vi "z_control_statemachine.vi"(4 "Kiz_down":sgl format="%#_13g", 6 "z_axis_params":T1={"TOL"=0.0, "ramp_rate"=-5e-06, "z_u_max"=5.0, "setpoint"=0.0, "Ki"=0.0, "Z_error_threshold"=0.0, "Z_settled_samples_threshold "=0, "z_UP"=1.5, "zup_N"=5000} {"ramp_rate" format="%#_4g"}, 7 "step_down":bool, 8 "step_down_frac":fxp<+,8,1>, 9 "init Z up":fxp<+/-,16,5>, 10 "State":i8, 11 "zerr(k)":fxp<+/-,16,5>) -> (3 "z-u(k)":fxp<+/-,16,5>)   [LabVIEW 2017]
uses:
  controls/z-axis-params_ssxy.ctl
  <vilib>/rvi/Emulation/niFpgaEmulationIsFPGAContextNoSignature.vi
  <vilib>/rvi/DataTransferAndStorage/Container/Common/niFpgaContainerGetUniqueNameForEmu.vi
  <vilib>/rvi/Memory/Memory_Emulation/niFpgaMemoryEmulationCacheClearOnFirstRun.vi
  <vilib>/rvi/Memory/Memory_Emulation/nirvimemoryEmulationManagerCache_MakeExclusive.vi
  <vilib>/rvi/Memory/Memory_Emulation/niFpgaMemoryEmulationValidateCache.vi
  <vilib>/rvi/Memory/Memory_Emulation/nirvimemoryEmulationManagerCache_InsertValue.vi
  <vilib>/Utility/error.llb/Clear Errors.vi
  <vilib>/rvi/Memory/Memory_Emulation/nirvimemoryEmulationManagerCache_ReleaseExclusive.vi
  <vilib>/rvi/Memory/Memory_Emulation/nirvimemoryEmulationManagerCache_GetValue.vi
  <vilib>/rvi/Memory/Memory_Emulation/nirvimemoryEmulationManagerCache_SetValue.vi
  <vilib>/rvi/Emulation/niFpgaProcessEmulError.vi
  <vilib>/rvi/Emulation/niFpgaSctlEmulationGetInTimedLoop.vi
  <vilib>/rvi/DataTransferAndStorage/Container/XNode/niFpgaContainer.xnode
  <vilib>/rvi/DataTransferAndStorage/Register/Emulation/niFpgaRegisterEmulation.vi
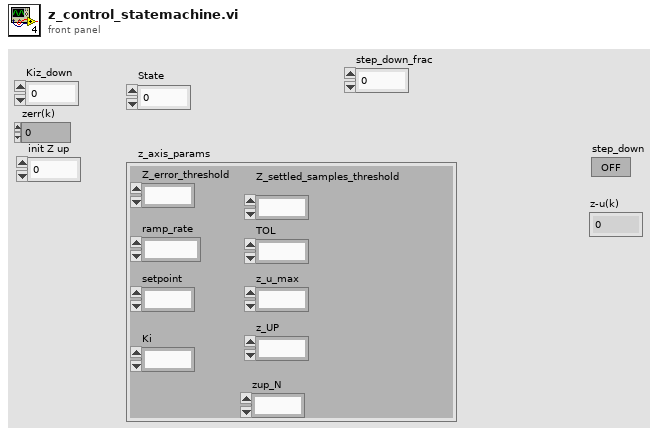
[diagram p1: front panel]
types:
  T1 = typedef "z-axis-params_ssxy.ctl" = cluster{"TOL":fxp<+/-,16,2>, "ramp_rate":sgl, "z_u_max":fxp<+/-,16,5>, "setpoint":fxp<+/-,16,5>, "Ki":fxp<+,16,1>, "Z_error_threshold":fxp<+/-,16,5>, "Z_settled_samples_threshold ":i16, "z_UP":fxp<+/-,16,5>, "zup_N":i16}
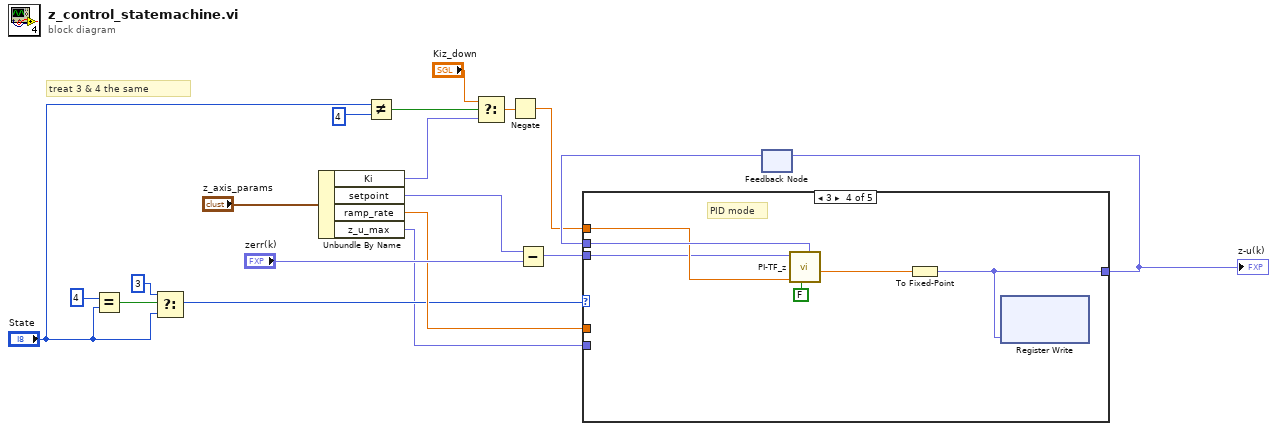
[diagram p0: block diagram]
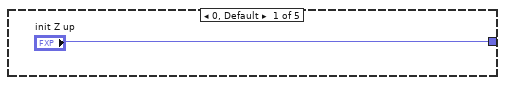
[diagram p2: hidden frame]
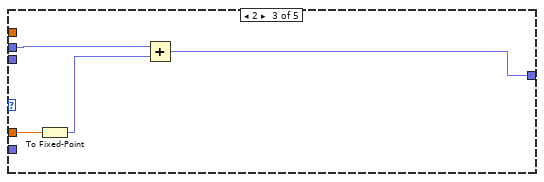
[diagram p4: hidden frame]
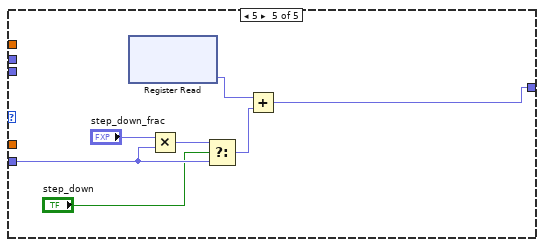
[diagram p5: hidden frame]
diagram:
  # "treat 3 & 4 the same"
  n1 = Equal?(x=i8 4 ("y"), y="State") -> (x = y?=w9:bool)
  n2 = Select(t=i8 3 ("y"), s=w9, f="State") -> (s? t:f=w7:i8)
  n3 = Unbundle By Name("z_axis_params") -> ("Ki"=w2:fxp<+,16,1>, "setpoint"=w3:fxp<+/-,16,5>, "ramp_rate"=w10:sgl, "z_u_max"=w1:fxp<+/-,16,5>)
  n4 = Not Equal?(x="State", y=i8 4) -> (x != y?=w18:bool)
  n5 = Select(t="Kiz_down", s=w18, f=w2) -> (s? t:f=w17:sgl)
  n6 = Negate(x=w17) -> (-x=w12:sgl)
  n7 = Subtract(x=w3, y="zerr(k)") -> (x-y=w11:fxp<+/-,17,6>)
  n8 = feedback #1() -> (w13:fxp<+/-,25,7>)  [unwired: 1 in]
  n9 = case shown="3" w7 {
    tunnel: ["init Z up" w21 w24 w26 w34] -> w6
    tunnel: w13 -> [_ w21 w22 w30 _]
    tunnel: w12 -> [_ _ _ w29 _]
    tunnel: w11 -> [_ _ _ w28 _]
    tunnel: w10 -> [_ _ w25 _ _]
    tunnel: w1 -> [_ _ _ _ w33]
    frame 0, Default {
    }
    frame 1 {
      # "XY-move, hold still, for now"
    }
    frame 2 {
      n10 = To Fixed-Point(number=w25) -> (fixed-point=w23:fxp<+/-,16,5>)  [unwired: 1 in]
      n11 = Add(x=w22, y=w23) -> (x+y=w24:fxp<+/-,16,5>)
    }
    frame 3 {
      # "PID mode"
      n12 = call "PI-TF_z.vi"("u(k-1)"=w30, "reset"=FALSE, "Ki"=w29, "e(k)"=w28) -> ("u(k)"=w27:sgl)  [unwired: 7 in]
      n13 = To Fixed-Point(number=w27) -> (fixed-point=w26:fxp<+/-,16,5>)  [unwired: 1 in]
      n14 = xnode ("Register Write")("Data"=w26) -> ()  [unwired: 1 in, 1 out]
    }
    frame 5 {
      n15 = xnode ("Register Read")() -> ("Data"=w35:fxp<+/-,16,5>)  [unwired: 1 in, 1 out]
      n16 = Multiply(x="step_down_frac", y=w33) -> (x*y=w38:fxp<+/-,24,6>)
      n17 = Select(t=w38, s="step_down", f=w33) -> (s? t:f=w36:fxp<+/-,24,6>)
      n18 = Add(x=w35, y=w36) -> (x+y=w34:fxp<+/-,25,7>)
    }
  }
  "z-u(k)" <- w6
  n19 = feedback-in #1(w6) -> ()
